vi "Simple Network Streams - Host.vi"() -> ()   [LabVIEW 2015]
doc: "Demonstrates how to use network streams to pass data and commands between two running VIs. It displays waveform data that is received from the target VI and sends commands to update the frequency of the generated signal."
uses:
  Control 1.ctl
  <vilib>/Platform/TimedLoop/XDataNode/timing_clust.ctl
  <vilib>/Platform/TimedLoop/XDataNode/nitl_modes.ctl
  <vilib>/Platform/TimedLoop/XDataNode/wakeup.ctl
  <vilib>/platform/TimedLoop/XDataNode/XDataNode.xnode
  <vilib>/ErrorRing/Error Ring.xnode
  <vilib>/Platform/TimedLoop/XDataNode/XDNodeRunTimeDep.lvlib
panel:
  out "Time":u32
  out "output cluster":T1
  in  "Target IP Address":string="192.168.150.78"
  # "Overview: Demonstrates how to use Network Streams to pass data and commands between two running VIs.\nRequirements: Windows\nInstructions:\n1. Make sure Simple Network Streams - Target.vi is already running.\n2. Run this VI.\n3. Change the Frequency value and observe the change in data that results from sending the new frequency value to the Target VI.\n4. Change the Read Speed value in this VI, and the Write Speed value in the Target VI, and observe the resulting values of Available Elements to Read and Available Elements to Write.\n5. Click Stop to stop the VI."
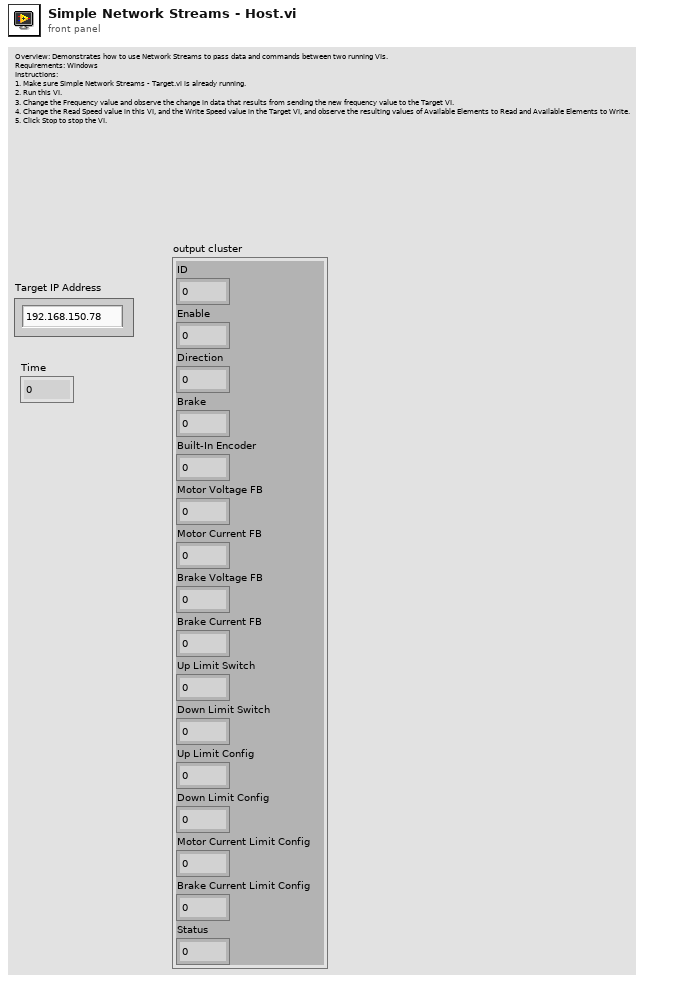
[diagram p1: front panel]
types:
  T1 = cluster{"ID":dbl, "Enable":dbl, "Direction":dbl, "Brake":dbl, "Built-In Encoder":dbl, "Motor Voltage FB":dbl, "Motor Current FB":dbl, "Brake Voltage FB":dbl, "Brake Current FB":dbl, "Up Limit Switch":dbl, "Down Limit Switch":dbl, "Up Limit Config":dbl, "Down Limit Config":dbl, "Motor Current Limit Config":dbl, "Brake Current Limit Config":dbl, "Status":dbl}
  T2 = typedef "Control 1.ctl" = cluster{"ID":dbl, "Enable":dbl, "Direction":dbl, "Brake":dbl, "Built-In Encoder":dbl, "Motor Voltage FB":dbl, "Motor Current FB":dbl, "Brake Voltage FB":dbl, "Brake Current FB":dbl, "Up Limit Switch":dbl, "Down Limit Switch":dbl, "Up Limit Config":dbl, "Down Limit Config":dbl, "Motor Current Limit Config":dbl, "Brake Current Limit Config":dbl, "Status":dbl}
  T3 = typedef "XDNodeRunTimeDep.lvlib/timing_clust.ctl" = cluster{"Expected End [f-1]":u64, "Actual End [f-1]":u64, "Finished Late? [f-1]":bool, "Expected End [i-1]":u64, "Actual End [i-1]":u64, "Finished Late? [i-1]":bool, "Expected Start [i]":u64, "Actual Start [i]":u64, "Expected Start [f]":u64, "Actual Start [f]":u64, "Source Name":string, "Structure Name":string, "Period":i64, "Deadline":i64, "Offset":i64, "Start":i64, "Priority":i32, "Timeout":i32, "Mode":T4, "Wakeup Reason":T5, "Error":errorcluster, "Source Type":string, "Secondary Source Type":string, "Global End Time":u64, "Global Start Time":u64, "Frame Duration":u64, "Iteration Duration":u64, "Assigned CPU":i32, "I/O Scan Engine Mode":u32}
  T4 = typedef "XDNodeRunTimeDep.lvlib/nitl_modes.ctl" = enum32{"No Change", "Process missed periods, maintain original phase", "Discard missed periods, maintain original phase", "Process missed periods, ignore original phase", "Discard missed periods, ignore original phase"}
  T5 = typedef "XDNodeRunTimeDep.lvlib/wakeup.ctl" = enum32{"Normal", "Aborted", "Asynchronous wakeup", "Timing source error", "Timed loop error", "Timeout"}
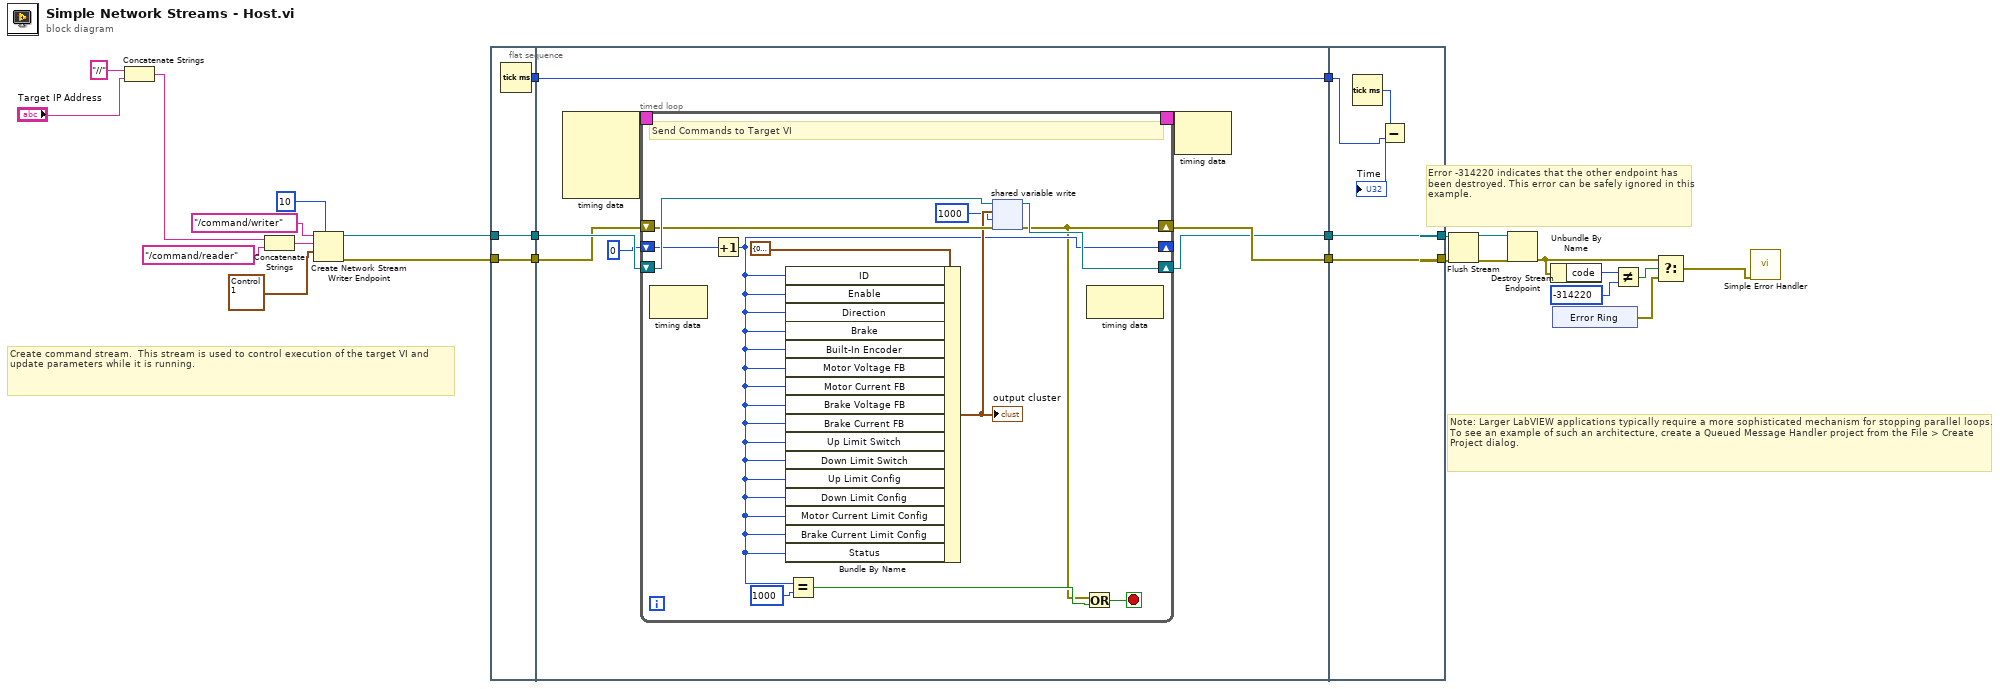
[diagram p0: block diagram]
diagram:
  # "Note: Larger LabVIEW applications typically require a more sophisticated mechanism for stopping parallel loops. To see an example of such an architecture, create a Queued Message Handler project from the File > Create Project dialog."
  # "Error -314220 indicates that the other endpoint has been destroyed. This error can be safely ignored in this example."
  # "Create command stream.  This stream is used to control execution of the target VI and update parameters while it is running."
  n1 = Concatenate Strings("//" ("reader url"), "Target IP Address") -> (w23:string)
  n2 = Concatenate Strings(w23, "/command/reader" ("reader url")) -> (w24:string)
  n3 = Create Network Stream Writer Endpoint(7:10 ("writer buffer size"), 9:T2 {"ID"=0.0, "Enable"=0.0, "Direction"=0.0, "Brake"=0.0, "Built-In Encoder"=0.0, "Motor Voltage FB"=0.0, "Motor Current FB"=0.0, "Brake Voltage FB"=0.0, "Brake Current FB"=0.0, "Up Limit Switch"=0.0, "Down Limit Switch"=0.0, "Up Limit Config"=0.0, "Down Limit Config"=0.0, "Motor Current Limit Config"=0.0, "Brake Current Limit Config"=0.0, "Status"=0.0} ("output cluster"), 10:w24, 11:"/command/writer" ("writer name")) -> (0:w19:errorcluster, 3:w20:refnum<k21>)  [unwired: 3 in]
  n4 = flat-sequence {
    tunnel: w19 -> [w28]
    tunnel: w20 -> [w29]
    tunnel: [w29] -> w6
    tunnel: [w28] -> w5
    tunnel: [w27] -> w1
    tunnel: w6 -> [w35]
    tunnel: w5 -> [w34]
    tunnel: [w33] -> w4
    tunnel: [w32] -> w3
    tunnel: [w30] -> w2
    tunnel: w1 -> [w30]
    tunnel: [w57] -> w7
    tunnel: [w58] -> w10
    tunnel: w4 -> [w58]
    tunnel: w3 -> [w57]
    tunnel: w2 -> [w55]
    frame #0 {
      n5 = Tick Count (ms)() -> (millisecond timer value=w27:u32)
    }
    frame #1 {
      n6 = node-c288() -> (w37:T3)  [unwired: 4 in]
      n7 = timed-loop "Host->Target Command Writer" {
        shift-right: [w38] -> w33
        shift-left: w34 -> [w48]
        shift-right: [w47] -> w32
        shift-left: w35 -> [w49]
        shift-right: [w42] -> _
        shift-left: 0 -> [w44]
        timing: w37 -> [_]
        timing-out: [_] -> w36
        stop <- w40 stop-if-true
        # "Send Commands to Target VI"
        n8 = node-c288() -> ()  [unwired: 1 in, 1 out]
        n9 = Increment(x=w44) -> (x+1=w42:i32)
        n10 = Bundle By Name(cluster=T1 {"ID"=0.0, "Enable"=0.0, "Direction"=0.0, "Brake"=0.0, "Built-In Encoder"=0.0, "Motor Voltage FB"=0.0, "Motor Current FB"=0.0, "Brake Voltage FB"=0.0, "Brake Current FB"=0.0, "Up Limit Switch"=0.0, "Down Limit Switch"=0.0, "Up Limit Config"=0.0, "Down Limit Config"=0.0, "Motor Current Limit Config"=0.0, "Brake Current Limit Config"=0.0, "Status"=0.0} ("MirrorCoverMotor"), "ID"=w42, "Enable"=w42, "Direction"=w42, "Brake"=w42, "Built-In Encoder"=w42, "Motor Voltage FB"=w42, "Motor Current FB"=w42, "Brake Voltage FB"=w42, "Brake Current FB"=w42, "Up Limit Switch"=w42, "Down Limit Switch"=w42, "Up Limit Config"=w42, "Down Limit Config"=w42, "Motor Current Limit Config"=w42, "Brake Current Limit Config"=w42, "Status"=w42) -> (w45:T1)
        "output cluster" <- w45
        n11 = Equal?(x=w42, y=1000) -> (x = y?=w39:bool)
        n12 = shared-variable-write(w49, w48, w45, 1000) -> (w47:refnum<k21>, w38:errorcluster)  [unwired: 1 out]
        n13 = Or(x=w38, y=w39) -> (x .or. y?=w40:bool)
        n14 = node-c288() -> ()  [unwired: 1 in, 1 out]
      }
      n15 = node-c288(w36) -> ()  [unwired: 1 out]
    }
    frame #2 {
      n16 = Tick Count (ms)() -> (millisecond timer value=w56:u32)
      n17 = Subtract(x=w56, y=w55) -> (x-y=→"Time":u32)
    }
  }
  n18 = Flush Stream(8:w10, 11:w7) -> (0:w9:errorcluster, 3:w8:refnum<k21>)  [unwired: 2 in, 1 out]
  n19 = Destroy Stream Endpoint(8:w9, 11:w8) -> (0:w14:errorcluster)
  n20 = Unbundle By Name(w14) -> ("code"=w15:i32)
  n21 = xnode "Error Ring"() -> ("error out"=w18:errorcluster)
  n22 = Not Equal?(x=w15, y=-314220) -> (x != y?=w17:bool)
  n23 = Select(t=w14, s=w17, f=w18) -> (s? t:f=w13:errorcluster)
  n24 = call <vilib>:"Simple Error Handler.vi"("error in (no error)"=w13) -> ()  [unwired: 4 in, 5 out]
